vi "Rate_Sample.vi"(8 "Funk_pom":enum32{"F:1", "F:2"}(radio), 9 "Chart/Graph":bool, 10 "Czas_cyklu":dbl, 11 "ilosc_ai":dbl) -> (2 "Sample":i32, 3 "Rate":dbl)   [LabVIEW 2021]
panel:
  # "Funkcje pomiarowe"
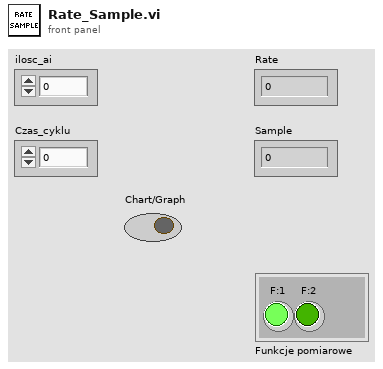
[diagram p1: front panel]
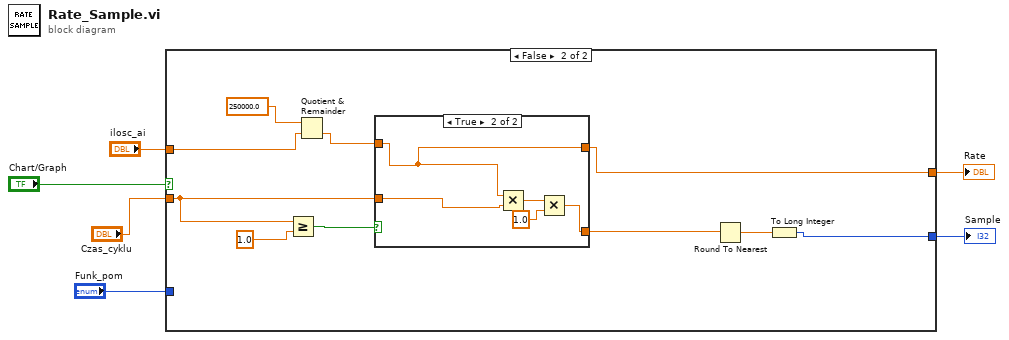
[diagram p0: block diagram]
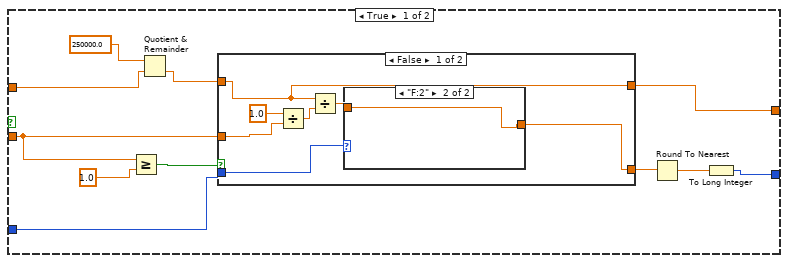
[diagram p2: hidden frame]
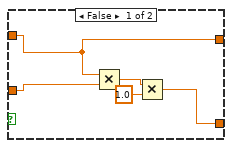
[diagram p6: hidden frame]
diagram:
  n1 = case shown="False" "Chart/Graph" {
    tunnel: "ilosc_ai" -> [w11 w35]
    tunnel: "Czas_cyklu" -> [w10 w34]
    tunnel: [w9 w33] -> w3
    tunnel: [w8 w32] -> w2
    tunnel: "Funk_pom" -> [w7 _]
    frame True {
      n2 = Greater Or Equal?(x=w10, y=1.0) -> (x >= y?=w16:bool)
      n3 = Quotient & Remainder(x=250000.0, y=w11) -> (floor(x/y)=w14:dbl)  [unwired: 1 out]
      n4 = case shown="False" w16 {
        tunnel: [w18 w28] -> w13
        tunnel: w10 -> [w23 _]
        tunnel: w14 -> [w20 w29]
        tunnel: [w20 w29] -> w9
        tunnel: w7 -> [w19 w27]
        frame False {
          n5 = Divide(x=1.0, y=w23) -> (x/y=w22:dbl)
          n6 = Divide(x=w20, y=w22) -> (x/y=w21:dbl)
          n7 = case shown="\"F:2\"" w19 {
            tunnel: w21 -> [w25 w26]
            tunnel: [w25 w26] -> w18
            frame "F:1" {
            }
            frame "F:2" {
            }
          }
        }
        frame True {
          n8 = case shown="\"F:1\"" w27 {
            tunnel: w29 -> [w30 w31]
            tunnel: [w30 w31] -> w28
            frame "F:1" {
            }
            frame "F:2" {
            }
          }
        }
      }
      n9 = Round To Nearest(number=w13) -> (nearest integer value=w12:dbl)
      n10 = To Long Integer(number=w12) -> (32bit integer=w8:i32)
    }
    frame False {
      n11 = Greater Or Equal?(x=w34, y=1.0) -> (x >= y?=w40:bool)
      n12 = Quotient & Remainder(x=250000.0, y=w35) -> (floor(x/y)=w38:dbl)  [unwired: 1 out]
      n13 = case shown="True" w40 {
        tunnel: [w42 w48] -> w37
        tunnel: w34 -> [w45 w50]
        tunnel: w38 -> [w46 w51]
        tunnel: [w46 w51] -> w33
        frame False {
          n14 = Multiply(x=w46, y=w45) -> (x*y=w44:dbl)
          n15 = Multiply(x=w44, y=1.0) -> (x*y=w42:dbl)
        }
        frame True {
          n16 = Multiply(x=w51, y=w50) -> (x*y=w49:dbl)
          n17 = Multiply(x=w49, y=1.0) -> (x*y=w48:dbl)
        }
      }
      n18 = Round To Nearest(number=w37) -> (nearest integer value=w36:dbl)
      n19 = To Long Integer(number=w36) -> (32bit integer=w32:i32)
    }
  }
  "Rate" <- w3
  "Sample" <- w2
